vi "SetSystemTimeZone_UTCOffset.vi"(0 "Requested UTC Offset":dbl, 11 "Error in":errorcluster caption="Error in (no error)") -> (4 "UTC Offset Set":dbl, 15 "Error out":errorcluster)   [LabVIEW 2017, in "GPTiming.lvlib"]
doc: "Sets the timezone closest possible to <B>Requested UTC Offset</B> on the (Windows only) system.\n\nAs <B>Requested UTC Offset</B> is a floating point number (since certain fractional hour timezones are defined), the actual <B>UTC Offset Set</B> is returned.\n\nThis VI runs only if there is no error on <B>Error in</B>.\n\nSteen Schmidt\nGPower\n4/2 2017"
uses:
  GPTiming.lvlib
  Error/GPError.lvlib
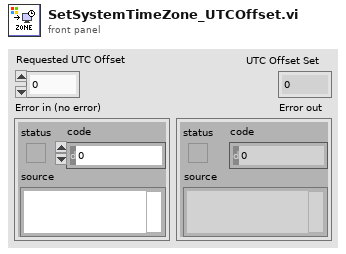
[diagram p1: front panel]
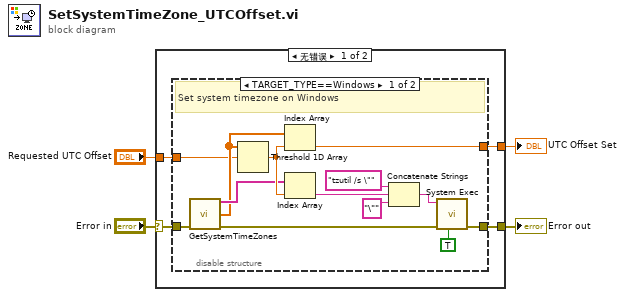
[diagram p0: block diagram]
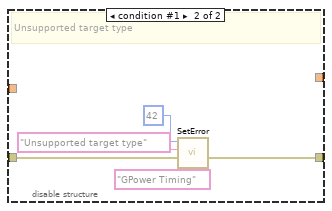
[diagram p2: hidden frame]
diagram:
  n1 = case shown="无错误" "Error in" {
    selector: "Error in" -> [w8 w27]
    tunnel: [w7 w27] -> w2
    tunnel: "Requested UTC Offset" -> [w6 _]
    tunnel: [w5 _] -> w1
    frame No Error {
      n2 = disable-structure shown="TARGET_TYPE==Windows" {
        disable-tunnel: w8 -> [w12 w24]
        disable-tunnel: [w9 w22] -> w7
        disable-tunnel: w6 -> [w11 _]
        disable-tunnel: [w10 _] -> w5
        frame condition #0 (active) {
          # "Set system timezone on Windows"
          n3 = call "GetSystemTimeZones.vi"("Error in"=w12) -> ("System Timezone Names"=w15:string[], "UTC Offsets"=w14:dbl[], "Error out"=w13:errorcluster)  [unwired: 11 in, 1 out]
          n4 = Threshold 1D Array(2:w11, 3:w14) -> (0:w17:dbl)  [unwired: 1 in]
          n5 = Index Array(array=w14, index=w17) -> (element=w10:dbl)
          n6 = Index Array(array=w15, index=w17) -> (element=w16:string)
          n7 = Concatenate Strings("tzutil /s \"" ("command line"), w16, "\"" ("command line")) -> (w21:string)
          n8 = call <vilib>:"System Exec.vi"("run minimized? (F)"=TRUE, "error in (no error)"=w13, "command line"=w21) -> ("error out"=w9:errorcluster)  [unwired: 5 in, 3 out]
        }
        frame condition #1 {
          # "Unsupported target type"
          n9 = call "SetError.vi"("Error label"="GPower Timing", "Error in"=w24, "Error description"="Unsupported target type", "Error code"=42) -> ("Error out"=w22:errorcluster)  [unwired: 7 in]
        }
      }
    }
    frame Error {
    }
  }
  "Error out" <- w2
  "UTC Offset Set" <- w1
